vi "ConfigureTargetRate.vi"(8 "error in (no error)":errorcluster, 10 "Target Rate in":dbl=100.0, 11 "absolute overridden system definition file in":path) -> (0 "error out":errorcluster, 3 "absolute overridden system definition file out":path)   [LabVIEW 2016, in "VeriStandTestCase.lvclass"]
uses:
  VeriStandTestCase.lvclass
  VeriStandTestUtilities/VeriStandTestUtilities.lvlib
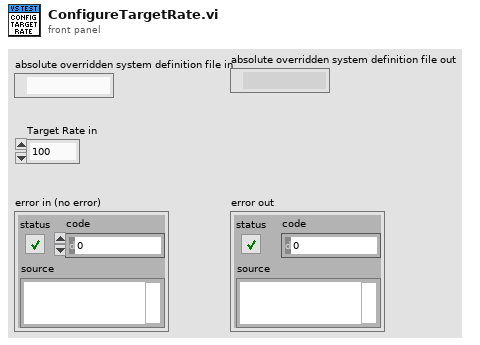
[diagram p1: front panel]
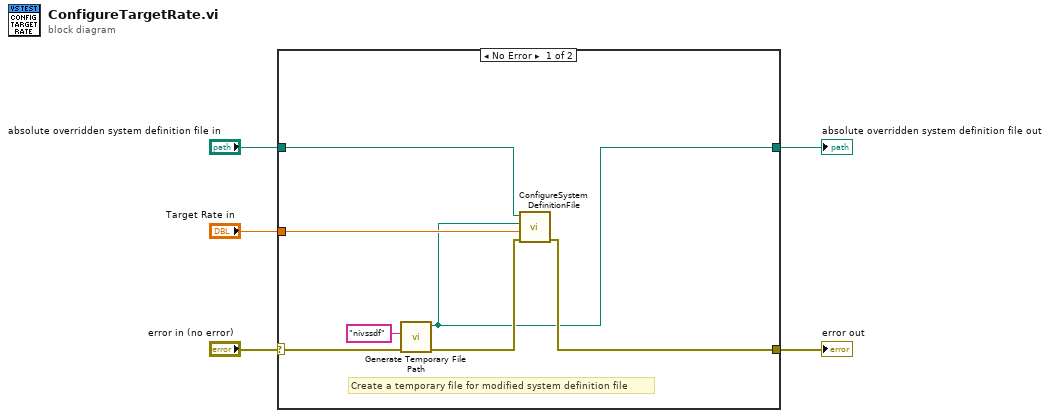
[diagram p0: block diagram]
diagram:
  n1 = case shown="No Error" "error in (no error)" {
    selector: "error in (no error)" -> [w10 w13]
    tunnel: [w12 w13] -> w4
    tunnel: "absolute overridden system definition file in" -> [w8 w14]
    tunnel: [w7 w14] -> w2
    tunnel: "Target Rate in" -> [w11 _]
    frame No Error {
      # "Create a temporary file for modified system definition file"
      n2 = call <vilib>:"Generate Temporary File Path.vi"("error in (no error)"=w10, "Temporary File Extension (tmp)"="nivssdf") -> ("error out"=w9:errorcluster, "Unique Temporary File Path"=w7:path)  [unwired: 8 in]
      n3 = call "ConfigureSystemDefinitionFile.vi"("error in (no error)"=w9, "Target Rate"=w11, "Destination System Definition File in"=w7, "Source System Definition File in"=w8) -> ("error out"=w12:errorcluster)  [unwired: 7 in]
    }
    frame Error {
    }
  }
  "error out" <- w4
  "absolute overridden system definition file out" <- w2
